vi "startup.vi"(8 "error in (no error)":errorcluster, 11 "WinX32Settings in":refnum<class "WinX32Settings.lvclass">) -> (0 "error out":errorcluster, 3 "WinX32Settings out":refnum<class "WinX32Settings.lvclass">)   [LabVIEW 2011, in "Tools.lvlib" / "Settings.lvlib" / "WinX32Settings.lvclass"]
uses:
  WinX32Settings.lvclass
  WinX32Settings.lvclass/WinX32Settings.ctl
  Filing/FileSystem/FileSystem.lvclass
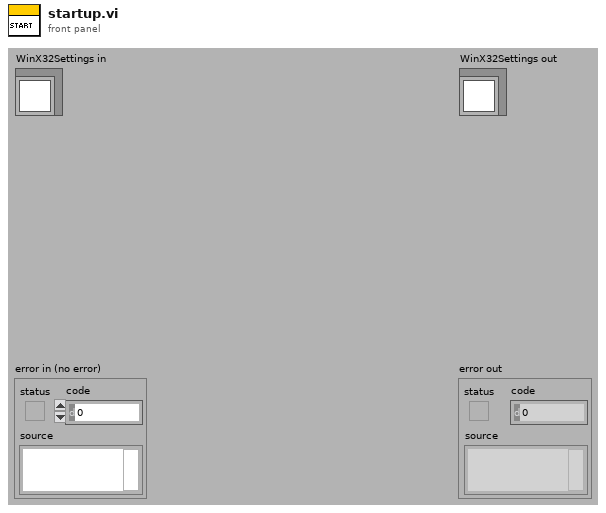
[diagram p1: front panel]
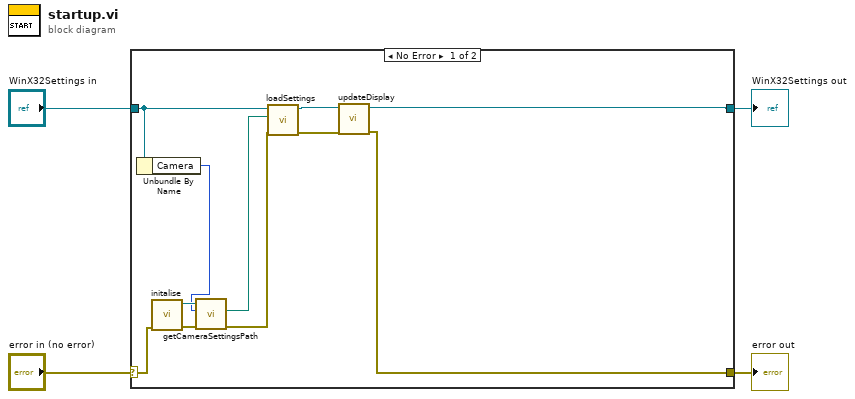
[diagram p0: block diagram]
diagram:
  n1 = case shown="No Error" "error in (no error)" {
    selector: "error in (no error)" -> [w13 w17]
    tunnel: [w8 w17] -> w3
    tunnel: [w7 w16] -> w1
    tunnel: "WinX32Settings in" -> [w6 w16]
    frame No Error {
      n2 = Unbundle By Name(w6) -> ("Camera"=w5:enum16{"Pixis", "ProEM", "PixelFly"})
      n3 = call "initalise.vi"("error in (no error)"=w13) -> ("error out"=w14:errorcluster, "FileSystem out"=w15:refnum<class "FileSystem.lvclass">)  [unwired: 9 in]
      n4 = call-dynamic "getCameraSettingsPath.vi"("error in (no error)"=w14, "Camera"=w5, "FileSystem.lvclass in"=w15) -> ("error out"=w11:errorcluster, "CameraSettingsPath"=w12:path)  [unwired: 6 in, 1 out]
      n5 = call-dynamic "loadSettings.vi"("error in (no error)"=w11, "Path"=w12, "WinX32Settings in"=w6) -> ("error out"=w9:errorcluster, "WinX32Settings out"=w10:refnum<class "WinX32Settings.lvclass">)  [unwired: 7 in]
      n6 = call "updateDisplay.vi"("error in (no error)"=w9, "WinX32Settings in"=w10) -> ("error out"=w8:errorcluster, "WinX32Settings out"=w7:refnum<class "WinX32Settings.lvclass">)  [unwired: 8 in]
    }
    frame Error {
    }
  }
  "error out" <- w3
  "WinX32Settings out" <- w1
